vi "MRate Decimation (FPGA).vi"() -> ()   [LabVIEW 2012]
uses:
  <vilib>/rvi/Emulation/niFpgaSctlEmulationGetInTimedLoop.vi
  <vilib>/rvi/DataTransferAndStorage/Container/Common/niFpgaContainerGetUniqueNameForEmu.vi
  <vilib>/rvi/FIFO/Fifo_Resource/nirvififoEmulationSetSize.vi
  <vilib>/rvi/Emulation/niFpgaSctlEmulationFifoFullMgr.vi
  <vilib>/rvi/errors/niFpgaSetErrorForExecOnDevCompSimple.vi
  <vilib>/rvi/eio/common/nirviEmuReportErrorAndStop.vi
  <vilib>/rvi/interface/RandomDataEmulation/nirviRandomDataFPGAFIFO.vi
  <vilib>/rvi/interface/RandomDataEmulation/niFpgaRandomDataHandleErrors.vi
  Instance           1 30Saved   MRateDecimation (FPGA) .vi
  <vilib>/rvi/eio/common/nirviEmuTemplateMethod_errors.vi
  <vilib>/rvi/Emulation/niFpgaSctlEmulationResourceMgr.vi
  <vilib>/rvi/DataTransferAndStorage/Container/XNode/niFpgaContainer.xnode
  <vilib>/rvi/FIFO/Fifo_Resource/nirvififoEmulationRead.vi
  <vilib>/rvi/interface/RandomDataEmulation/nirviRandomDataFpgaReadWriteTemplate.vi
  <vilib>/eio/EIONode/EIONode.xnode
  <vilib>/rvi/FIFO/Fifo_Resource/nirvififoEmulationWrite.vi
panel:
  out "Filtered Signals":u32(graph)
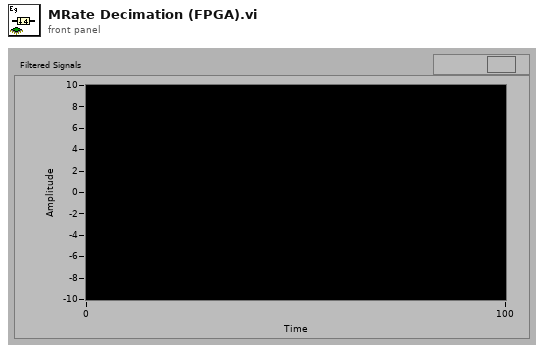
[diagram p1: front panel]
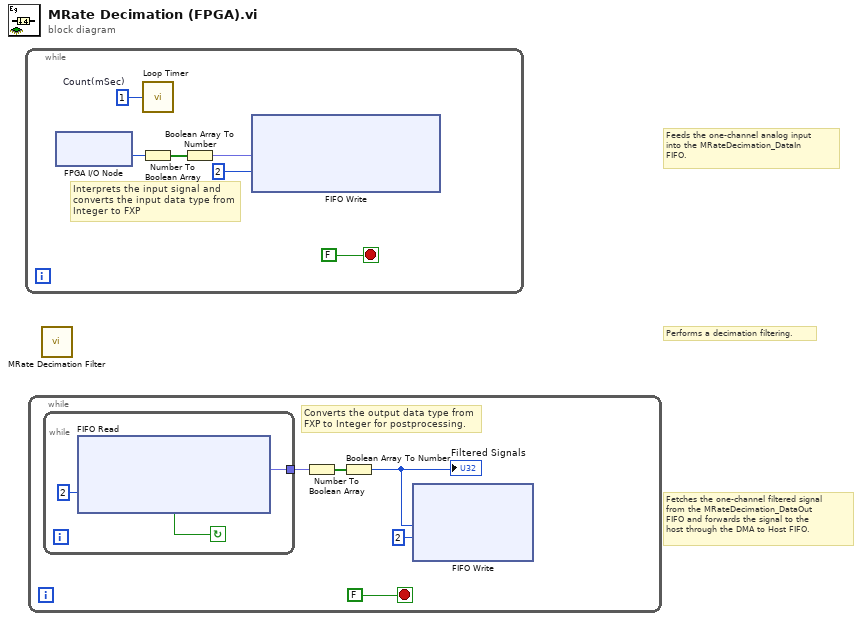
[diagram p0: block diagram]
diagram:
  # "Fetches the one-channel filtered signal\nfrom the MRateDecimation_DataOut\nFIFO and forwards the signal to the \nhost through the DMA to Host FIFO."
  # "Performs a decimation filtering."
  # "Feeds the one-channel analog input\ninto the MRateDecimation_DataIn\nFIFO."
  n1 = while {
    stop <- FALSE stop-if-true
    w5 = u16 1  # Count(mSec)
    # "Interprets the input signal and \nconverts the input data type from \nInteger to FXP"
    n2 = xnode "FPGA I/O Node"() -> ("AI0"=w2:i16)  [unwired: 1 in, 1 out]
    n3 = call "Loop Timer"("Count(mSec)"=w5) -> ()  [unwired: 1 out]
    n4 = Number To Boolean Array(number=w2) -> (Boolean array=w3:bool[])
    n5 = Boolean Array To Number(Boolean array=w3) -> (number=w1:fxp<+/-,16,1>)
    n6 = xnode ("FIFO Write")("Element"=w1, "Timeout"=2) -> ()  [unwired: 1 in, 2 out]
  }
  n7 = while {
    stop <- FALSE stop-if-true
    # "Converts the output data type from \nFXP to Integer for postprocessing."
    n8 = while {
      tunnel: [w12] -> w8
      stop <- w13 continue-if-true
      n9 = xnode ("FIFO Read")("Timeout"=2) -> ("Element"=w12:fxp<+/-,32,2>, "Timed Out?"=w13:bool)  [unwired: 1 in, 1 out]
    }
    n10 = Number To Boolean Array(number=w8) -> (Boolean array=w9:bool[])
    n11 = Boolean Array To Number(Boolean array=w9) -> (number=w7:u32)
    "Filtered Signals" <- w7
    n12 = xnode ("FIFO Write")("Element"=w7, "Timeout"=2) -> ()  [unwired: 1 in, 2 out]
  }
  n13 = call "MRate Decimation Filter.vi"() -> ()  [unwired: 1 out]
